vi "stop.vi"(8 "error in (no error)":errorcluster, 11 "TCPComEvents in":refnum<class "TCPComEvents.lvclass">) -> (0 "error out":errorcluster, 3 "TCPComEvents out":refnum<class "TCPComEvents.lvclass">)   [LabVIEW 2016, in "TCPComEvents.lvclass"]
uses:
  TCPComEvents.lvclass
  TCPComEvents.lvclass/TCPComEvents.ctl
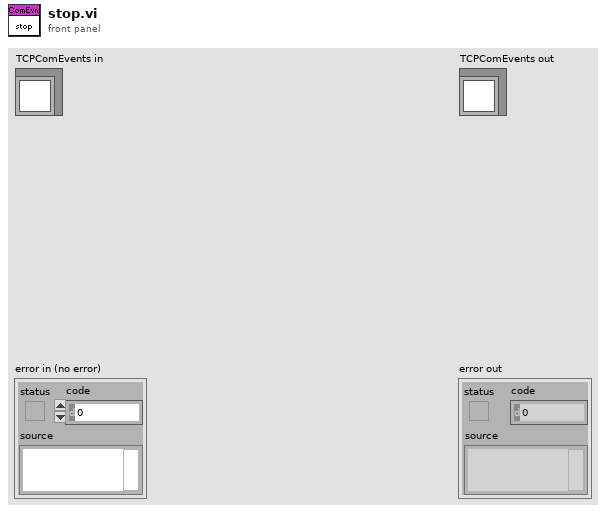
[diagram p1: front panel]
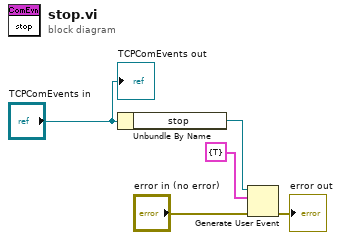
[diagram p0: block diagram]
diagram:
  n1 = Unbundle By Name("TCPComEvents in") -> ("stop"=w4:refnum<user-event>)
  n2 = Generate User Event(user event=w4, event data cluster=cluster{"stop":bool} {"stop"=TRUE} ("event data"), error in="error in (no error)") -> (error out=→"error out":errorcluster)  [unwired: 1 in, 1 out]
  "TCPComEvents out" <- "TCPComEvents in"
